vi "FindCorners.vi"() -> ()   [LabVIEW 2018]
panel:
  out "Image to process":picture
  out "Processed image":picture
  out "Error":errorcluster
  out "Corners marked in green":cluster{"X":u32, "Y":dbl}[](array[cluster])
  out "Corners marked in red":cluster{"X":u32, "Y":dbl}[](array[cluster])
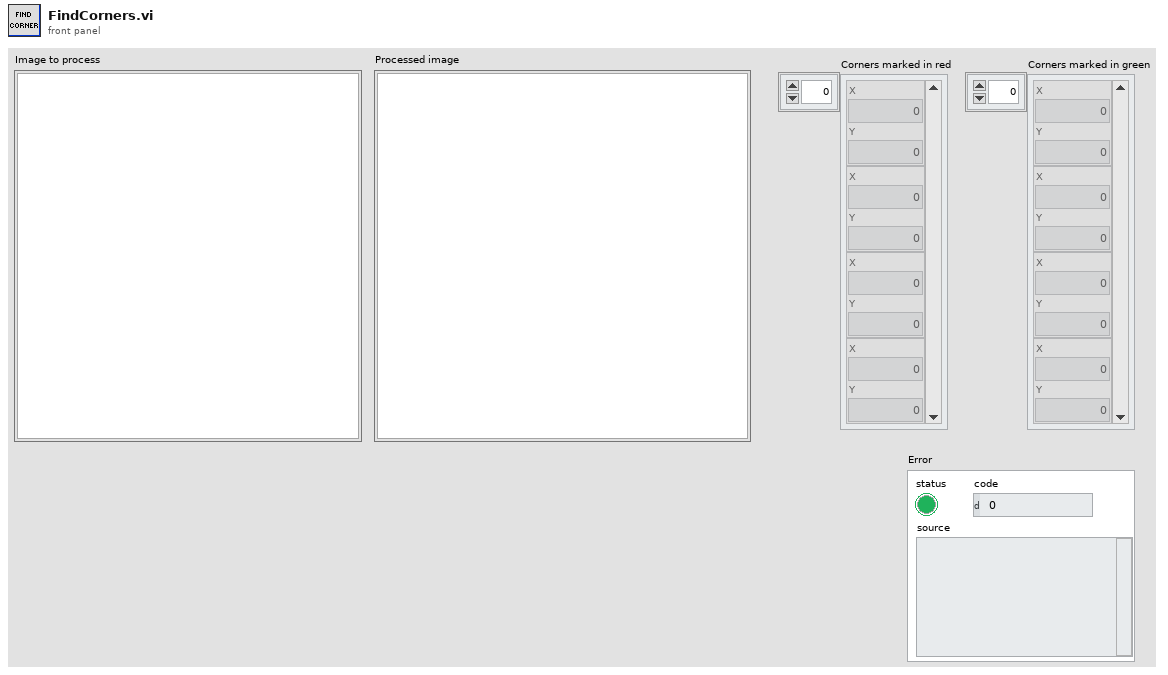
[diagram p1: front panel]
types:
  T1 = cluster{u32[][], cluster{u32, u32}[], cluster{u32, u32}[]}
  T2 = typedef "imagedata.ctl" = cluster{"image type":i32, "image depth":i32, "image":u8[], "mask":u8[], "colors":u32[], "Rectangle":cluster{"left":i16, "top":i16, "right":i16, "bottom":i16}}
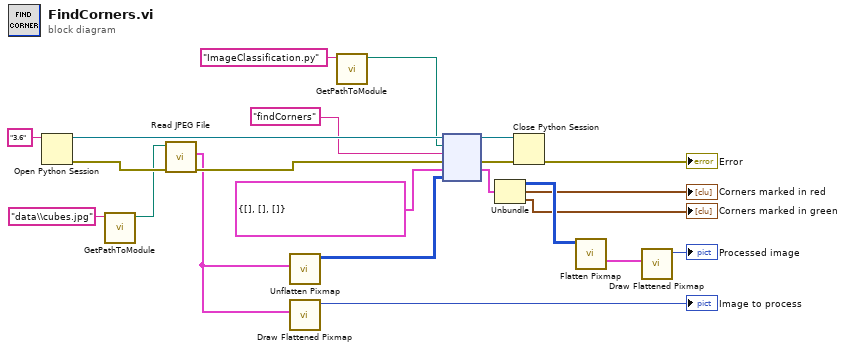
[diagram p0: block diagram]
diagram:
  n1 = Open Python Session(python version="3.6" ("Python version")) -> (session out=w22:refnum<k35>, error out=w16:errorcluster)  [unwired: 2 in]
  n2 = call "GetPathToModule.vi"("module name"="data\\cubes.jpg") -> ("path to module"=w1:path)  [unwired: 10 in]
  n3 = call <vilib>:"Read JPEG File.vi"("error in (no error)"=w16, "path to JPEG file"=w1) -> ("error out"=w15:errorcluster, "image data"=w13:T2)  [unwired: 7 in, 1 out]
  n4 = call <vilib>:"Unflatten Pixmap.vi"("image data"=w13) -> ("24-bit pixmap"=w10:u32[][])  [unwired: 4 in, 6 out]
  n5 = call <vilib>:"Draw Flattened Pixmap.vi"("image data"=w13) -> ("new picture"=→"Image to process":picture)  [unwired: 8 in]
  n6 = call "GetPathToModule.vi"("module name"="ImageClassification.py") -> ("path to module"=w4:path)  [unwired: 10 in]
  n7 = node(w22, w4, "findCorners" ("function name"), w15, T1 {[], [], []}, w10) -> (w21:refnum<k35>, w20:errorcluster, w8:T1)  [unwired: 1 in, 2 out]
  n8 = Unbundle(w8) -> (w7:u32[][], →"Corners marked in red":cluster{u32, u32}[], →"Corners marked in green":cluster{u32, u32}[])
  n9 = Close Python Session(session in=w21, error in=w20) -> (11:→"Error":errorcluster)
  n10 = call <vilib>:"Flatten Pixmap.vi"("24-bit pixmap"=w7) -> ("image data"=w18:T2)  [unwired: 10 in]
  n11 = call <vilib>:"Draw Flattened Pixmap.vi"("image data"=w18) -> ("new picture"=→"Processed image":picture)  [unwired: 8 in]
